vi "MenuDo.vi"(0 "LMenuCol in":refnum<class "ModeCol.lvclass">, 1 "Col Array Ref in":refnum<vi>, 2 "Layout Ring Refnum":refnum<vi>, 3 "Clipboard":refnum<vi>, 5 "ItemTag":string, 7 "VariableManagerRef":refnum<vi>, 9 "Table CtlRef In":refnum<vi>, 11 "error in (no error)":errorcluster, 12 "Cell Position":T1, 13 "ModeCol Index":i32=2, 14 "Table History ref":refnum<vi>) -> (4 "LMenuCol out":refnum<class "ModeCol.lvclass">, 6 "Col Array Ref out":refnum<vi>, 8 "Update HWI?":bool, 10 "Table CtlRef Out":refnum<vi>, 15 "error out":errorcluster)   [LabVIEW 2013, in "ModeCol.lvclass"]
doc: "Perform selected shortcut (right-click) menu actions for Mode column.\nThis VI is read-only w.r.t column data."
uses:
  ModeCol.lvclass
  <vilib>/Utility/miscctls.llb/LVRowAndColumnTypeDef.ctl
  TypeDefs/TableHistory.ctl
  TypeDefs/TableArray.ctl
  VariableManagerCodes/VariableManager/VariableManager.lvclass
  Column/Column.lvclass
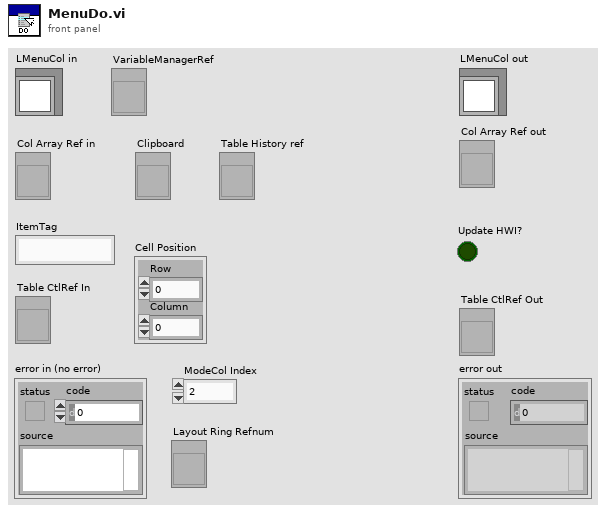
[diagram p1: front panel]
types:
  T1 = typedef "LVRowAndColumnTypeDef.ctl" = cluster{"Row":i32, "Column":i32}
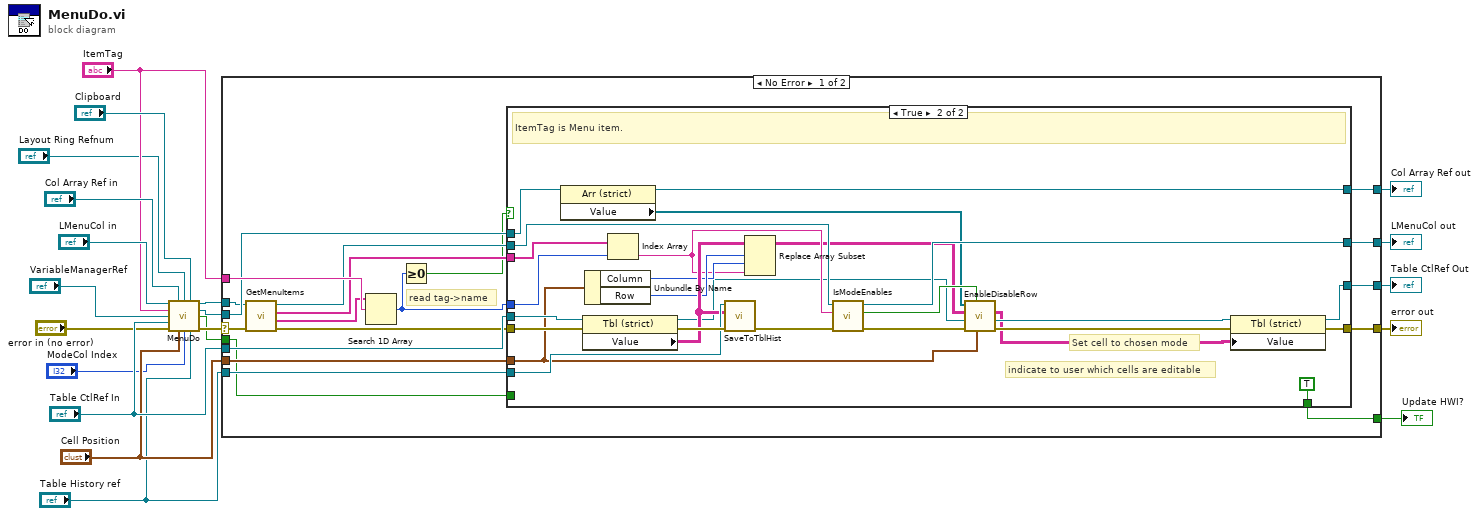
[diagram p0: block diagram]
diagram:
  n1 = call-parent "MenuDo.vi"("Column in"="LMenuCol in", "Col Array Ref in"="Col Array Ref in", "Layout Ring Refnum"="Layout Ring Refnum", "Clipboard"="Clipboard", "ItemTag"="ItemTag", "VariableManagerRef"="VariableManagerRef", "Table CtlRef In"="Table CtlRef In", "error in (no error)"="error in (no error)", "Cell Position"="Cell Position", "ModeCol Index"="ModeCol Index", "Table History ref"="Table History ref") -> ("Column out"=w9:refnum<class "ModeCol.lvclass">, "Col Array Ref out"=w8:refnum<vi>, "Update HWI?"=w2:bool, "error out"=w10:errorcluster)  [unwired: 1 out]
  n2 = case shown="No Error" w10 {
    selector: w10 -> [w27 w73]
    tunnel: [w39 w75] -> w20
    tunnel: [w38 w73] -> w19
    tunnel: [w37 w74] -> w18
    tunnel: [w36 w76] -> w17
    tunnel: "Table CtlRef In" -> [w35 w74]
    tunnel: "ItemTag" -> [w34 _]
    tunnel: w8 -> [w29 w76]
    tunnel: w9 -> [w28 w75]
    tunnel: "Cell Position" -> [w26 _]
    tunnel: "Table History ref" -> [w23 _]
    tunnel: w2 -> [w22 w72]
    tunnel: [w21 w72] -> w1
    frame No Error {
      # "read tag->name"
      n3 = call "GetMenuItems.vi"("error in (no error)"=w27, "ModeCol in"=w28) -> ("error out"=w33:errorcluster, "LMenu tags"=w32:string[], "LMenu names"=w31:string[], "ModeCol out"=w30:refnum<class "ModeCol.lvclass">)  [unwired: 6 in]
      n4 = Search 1D Array(1D array=w32, element=w34) -> (index of element=w24:i32)  [unwired: 1 in]
      n5 = Greater Or Equal To 0?(x=w24) -> (x >= 0?=w25:bool)
      n6 = case shown="True" w25 {
        tunnel: [w43 w71] -> w39
        tunnel: [w41 w49] -> w38
        tunnel: [w42 w50] -> w37
        tunnel: [w44 w59] -> w36
        tunnel: w35 -> [w42 w65]
        tunnel: w33 -> [w41 w64]
        tunnel: w24 -> [_ w70]
        tunnel: w31 -> [_ w69]
        tunnel: w30 -> [w43 w68]
        tunnel: w29 -> [w44 w61]
        tunnel: w26 -> [_ w58]
        tunnel: w23 -> [_ w62]
        tunnel: w22 -> [w40 _]
        tunnel: [w40 TRUE ("Update HWI?")] -> w21
        frame False {
          # "ItemTag not found!"
        }
        frame True {
          # "Set cell to chosen mode"
          # "indicate to user which cells are editable"
          # "ItemTag is Menu item."
          n7 = property class="Arr (strict)"(reference=w61) -> (reference out=w59:refnum<vi>, "Value"=w60:refnum<class "Column.lvclass">[])  [unwired: 1 in, 1 out]
          n8 = property class="Tbl (strict)"(reference=w65, error in=w64) -> (reference out=w53:refnum<vi>, error out=w63:errorcluster, "Value"=w57:string[][])
          n9 = Unbundle By Name(w58) -> ("Column"=w55:i32, "Row"=w56:i32)
          n10 = Index Array(array=w69, index=w70) -> (element=w54:string)
          n11 = call "SaveToTblHist.vi"("error in (no error)"=w63, "OldTable (reset)"=w57, "Table History ref"=w62) -> ("error out"=w47:errorcluster)  [unwired: 8 in]
          n12 = Replace Array Subset(array=w57, new element=w54, index (row)=w56, index (col)=w55) -> (w52:string[][])
          n13 = call "IsModeEnables.vi"("error in (no error)"=w47, "Mode value"=w54, "ModeCol in"=w68) -> ("error out"=w67:errorcluster, "Disable / Enable"=w66:bool, "ModeCol out"=w71:refnum<class "ModeCol.lvclass">)  [unwired: 6 in]
          n14 = call "EnableDisableRow.vi"("Cell Position"=w58, "Disable / Enable"=w66, "error in (no error)"=w67, "Table CtlRef In"=w53, "Table Data in"=w52, "Col Array in"=w60) -> ("error out"=w48:errorcluster, "Table CtlRef Out"=w51:refnum<vi>, "Table Data out"=w46:string[][])  [unwired: 3 in]
          n15 = property class="Tbl (strict)"(reference=w51, error in=w48, "Value"=w46) -> (reference out=w50:refnum<vi>, error out=w49:errorcluster)
        }
      }
    }
    frame Error {
    }
  }
  "error out" <- w19
  "LMenuCol out" <- w20
  "Table CtlRef Out" <- w18
  "Col Array Ref out" <- w17
  "Update HWI?" <- w1
